vi "DAQchannelStorage.vi"(3 "error in":errorcluster, 4 "DAQ Card/Channels":i32[](array[numeric]), 5 "Channel Settings":T1(array[cluster]), 6 "Tree DVR In":refnum<data-value>) -> (0 "error out":errorcluster)   [LabVIEW 2014]
doc: "Stores the 'DAQ' channel settings (for each DAQtive channel) to MDS+"
uses:
  <vilib>/MDSplus/Classes/Tree_Class/Tree.lvclass
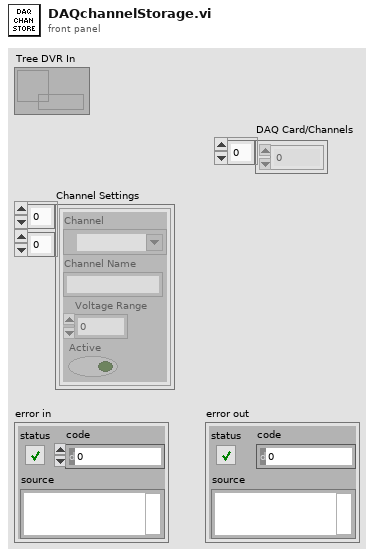
[diagram p1: front panel]
types:
  T1 = cluster{"Channel":tag, "Channel Name":string, "Voltage Range":dbl, "Active":bool}[][]
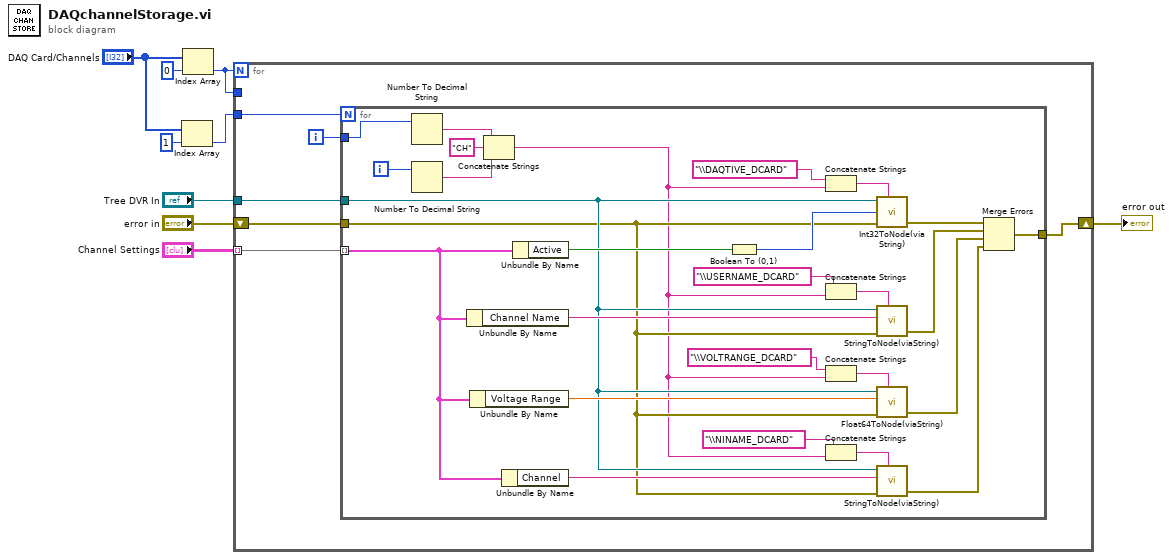
[diagram p0: block diagram]
diagram:
  n1 = Index Array(array="DAQ Card/Channels", index=1) -> (element=w2:i32)
  n2 = Index Array(array="DAQ Card/Channels", index=0) -> (element=w1:i32)
  n3 = for {
    N: w1 -> [_]
    shift-right: [w14] -> w6
    shift-left: "error in" -> [w12]
    tunnel: "Channel Settings" -> [w13] mode=indexing
    tunnel: "Tree DVR In" -> [w15]
    tunnel: w2 -> [w11]
    tunnel: w1 -> [_]
    i -> [w10]
    n4 = for {
      N: w11 -> [_]
      tunnel: w13 -> [w26] mode=indexing
      tunnel: w12 -> [w30]
      tunnel: w15 -> [w31]
      tunnel: [w28] -> w14
      tunnel: w10 -> [w19]
      i -> [w18]
      n5 = Number To Decimal String(number=w19) -> (decimal integer string=w21:string)  [unwired: 1 in]
      n6 = Number To Decimal String(number=w18) -> (decimal integer string=w20:string)  [unwired: 1 in]
      n7 = Unbundle By Name(w26) -> ("Channel Name"=w37:string)
      n8 = Unbundle By Name(w26) -> ("Voltage Range"=w34:dbl)
      n9 = Concatenate Strings(w21, "CH" ("string"), w20) -> (w22:string)
      n10 = Unbundle By Name(w26) -> ("Channel"=w32:tag)
      n11 = Unbundle By Name(w26) -> ("Active"=w40:bool)
      n12 = Boolean To (0,1)(Boolean=w40) -> (0, 1=w42:i16)
      n13 = Concatenate Strings("\\DAQTIVE_DCARD" ("string"), w22) -> (w41:string)
      n14 = Concatenate Strings("\\USERNAME_DCARD" ("string"), w22) -> (w38:string)
      n15 = Concatenate Strings("\\VOLTRANGE_DCARD" ("string"), w22) -> (w35:string)
      n16 = Concatenate Strings("\\NINAME_DCARD" ("string"), w22) -> (w17:string)
      n17 = call "Int32ToNode(viaString).vi"("Tree DVR in"=w31, "I32 in"=w42, "error in (no error)"=w30, "NodePath"=w41) -> ("error out"=w39:errorcluster)  [unwired: 3 in]
      n18 = call "StringToNode(viaString).vi"("Tree DVR in"=w31, "String value in"=w37, "error in (no error)"=w30, "NodePath"=w38) -> ("error out"=w36:errorcluster)  [unwired: 3 in]
      n19 = call "Float64ToNode(viaString).vi"("Tree DVR in"=w31, "DBL in"=w34, "error in"=w30, "NodePath"=w35) -> ("error out"=w33:errorcluster)  [unwired: 3 in]
      n20 = call "StringToNode(viaString).vi"("Tree DVR in"=w31, "String value in"=w32, "error in (no error)"=w30, "NodePath"=w17) -> ("error out"=w29:errorcluster)  [unwired: 3 in]
      n21 = Merge Errors(w39, w36, w33, w29) -> (w28:errorcluster)
    }
  }
  "error out" <- w6
